vi "Climb Functions.vi"(6 "Elevator Slow Velocity":dbl=400.0, 9 "Elevator Slow Acceleration":dbl=800.0, 10 "POVs":i16[](array[numeric]), 11 "Buttons":bool[](array[boolean])) -> ()   [LabVIEW 2019]
uses:
  Typedef/XBox Buttons.ctl
  <vilib>/Rock Robotics/WPI/Solenoid/WPI_SolenoidValue.ctl
  <vilib>/Rock Robotics/WPI/ThirdParty/REV Robotics/SPARK MAX/Typedef/Spark MAX Idle Mode.ctl
  <vilib>/Rock Robotics/WPI/Solenoid/WPI_SolenoidSetEnum.vi
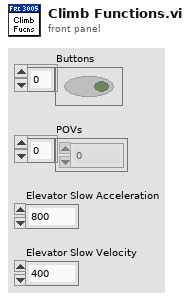
[diagram p1: front panel]
types:
  T1 = typedef "XBox Buttons.ctl" = enum16{"A", "B", "X", "Y", "Left Bumper", "Right Bumper", "Back", "Start", "Left Joystick", "Right Joystick"}
  T2 = typedef "Spark MAX Idle Mode.ctl" = enum16{"Coast", "Brake"}
  T3 = typedef "SPARKMAX6Motor.ctl" = cluster{"FrontLeftMaster":T4, "FrontLeftSlave1":T4, "FrontLeftSlave2":T4, "FrontRightMaster":T4, "FrontRightSlave1":T4, "FrontRightSlave2":T4}
  T4 = typedef "WPI_MotorControlDeviceRef.ctl" = cluster{"DeviceStatus":errorcluster, "Type":T5, "PWM":cluster{"PWM Channel":T6, "DeadBand":T7}, "CAN":cluster{"Device Number":u8, "SetOutput VI Ref":variant, "GetOutput VI Ref":variant, "Enable VI Ref":variant, "Disable VI Ref":variant, "Data":variant}, "Invert":bool, "DIO PWM":cluster{"PWM \"Enable\" Channel":T6, "DIOChannel":T8, "PWM Rate":dbl}}
  T5 = typedef "WPI_MotorControlType.ctl" = enum16{"PWM", "CAN", "DIO PWM"}
  T6 = typedef "FPGA_DIOPWMChannel.ctl" = enum8{"PWM 0", "PWM 1", "PWM 2", "PWM 3", "PWM 4", "PWM 5", "PWM 6", "PWM 7", "PWM 8", "PWM 9", "PWM MXP 0", "PWM MXP 1", "PWM MXP 2", "PWM MXP 3", "PWM MXP 4", "PWM MXP 5", "PWM MXP 6", "PWM MXP 7", "PWM MXP 8", "PWM MXP 9", "Invalid"}
  T7 = typedef "WPI_PWMDeadband.ctl" = cluster{"Name":string, "maxPositivePwm":i32, "minPositivePwm":i32, "centerPwm":i32, "maxNegativePwm":i32, "minNegativePwm":i32, "angularRange":u16}
  T8 = typedef "FPGA_DIOChannel.ctl" = enum8{"DIO 0", "DIO 1", "DIO 2", "DIO 3", "DIO 4", "DIO 5", "DIO 6", "DIO 7", "DIO 8", "DIO 9", "DIO MXP 0", "DIO MXP 1", "DIO MXP 2", "DIO MXP 3", "DIO MXP 4", "DIO MXP 5", "DIO MXP 6", "DIO MXP 7", "DIO MXP 8", "DIO MXP 9", "DIO MXP 10", "DIO MXP 11", "DIO MXP 12", "DIO MXP 13", "DIO MXP 14", "DIO MXP 15", "SPI Port CS1", "SPI Port CS2", "SPI Port CS3", "SPI Port MISO", "SPI Port MOSI", "Invalid"}
  T9 = typedef "WPI_SolenoidValue.ctl" = enum16{"Off", "On", "Forward", "Reverse"}
  T10 = typedef "WPI_SolenoidDevRef.ctl" = cluster{"DevStatus":errorcluster, "Pneumatics Control Module":u8, "Forward Solenoid Channel":T11, "Reverse Solenoid Channel":T11}
  T11 = typedef "WPI_SolenoidChannel.ctl" = enum8{"Solenoid 0", "Solenoid 1", "Solenoid 2", "Solenoid 3", "Solenoid 4", "Solenoid 5", "Solenoid 6", "Solenoid 7", "Invalid"}
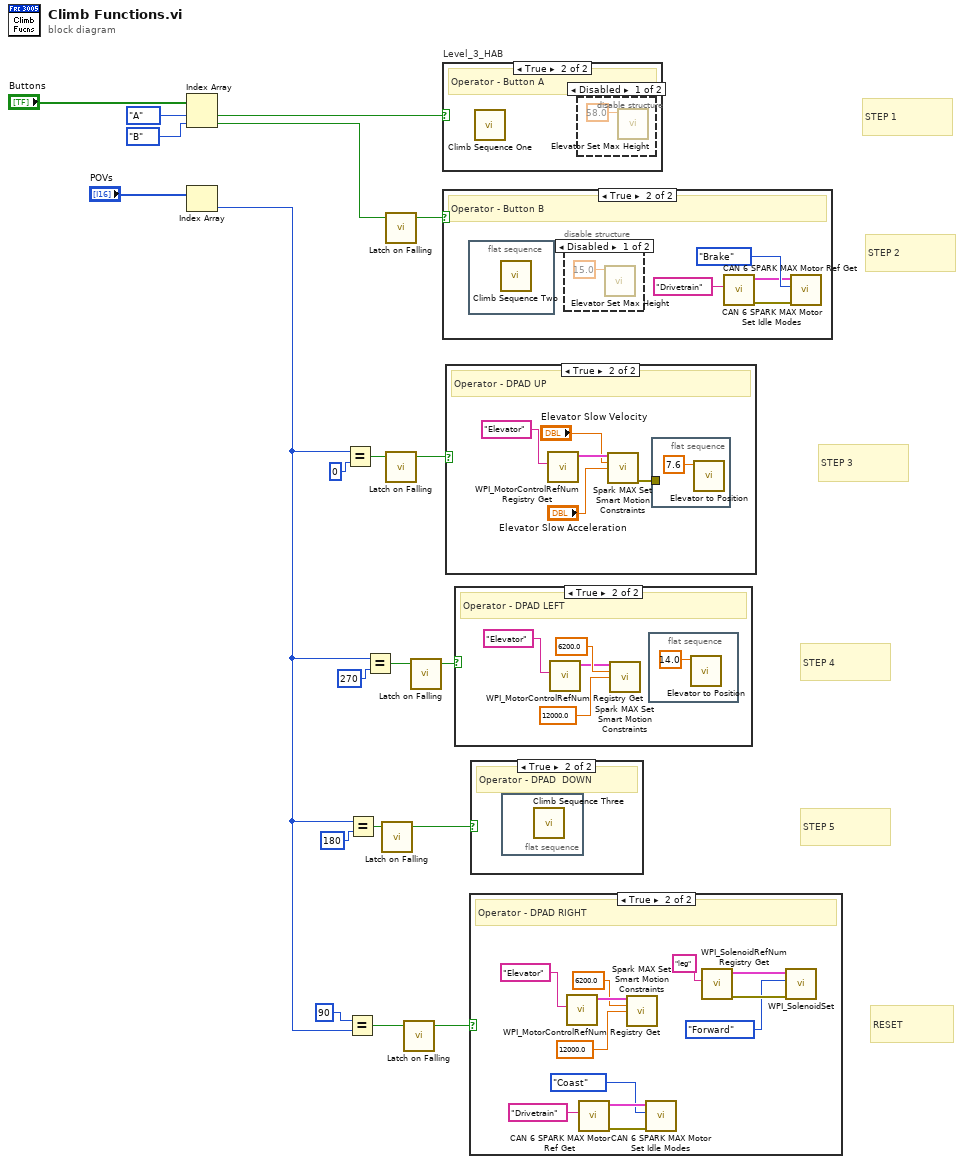
[diagram p0: block diagram]
diagram:
  # "RESET"
  # "STEP 5"
  # "STEP 4"
  # "STEP 3"
  # "STEP 2"
  # "STEP 1"
  n1 = Index Array(array="Buttons", index #1=XBox_Buttons."A" ("Enum"), index #2=XBox_Buttons."B" ("Enum")) -> (element #1=w20:bool, element #2=w19:bool)
  n2 = Index Array(array="POVs") -> (element=w15:i16)  [unwired: 1 in]
  n3 = Equal?(x=w15, y=i16 0 ("element")) -> (x = y?=w6:bool)
  n4 = Equal?(x=i16 90 ("element"), y=w15) -> (x = y?=w10:bool)
  n5 = Equal?(x=w15, y=i16 180 ("element")) -> (x = y?=w5:bool)
  n6 = Equal?(x=w15, y=i16 270 ("element")) -> (x = y?=w13:bool)
  n7 = call "Latch on Falling.vi"("Boolean in"=w5) -> ("Boolean out"=w2:bool)  [unwired: 4 in]
  n8 = call "Latch on Falling.vi"("Boolean in"=w19) -> ("Boolean out"=w3:bool)  [unwired: 4 in]
  n9 = call "Latch on Falling.vi"("Boolean in"=w6) -> ("Boolean out"=w8:bool)  [unwired: 4 in]
  n10 = call "Latch on Falling.vi"("Boolean in"=w10) -> ("Boolean out"=w11:bool)  [unwired: 4 in]
  n11 = call "Latch on Falling.vi"("Boolean in"=w13) -> ("Boolean out"=w14:bool)  [unwired: 4 in]
  n12 = case "Level_3_HAB" shown="True" w20 {
    frame False {
    }
    frame True {
      # "Operator - Button A"
      n13 = call "Climb Sequence One.vi"() -> ()  [unwired: 11 in, 1 out]
      n14 = disable-structure shown="Disabled" {
        frame Disabled {
          n15 = call "Elevator Set Max Height.vi"("Setpoint"=58.0) -> ()  [unwired: 10 in, 1 out]
        }
        frame Enabled {
        }
      }
    }
  }
  n16 = case shown="True" w3 {
    frame False {
    }
    frame True {
      # "Operator - Button B"
      n17 = flat-sequence {
        frame #0 {
          n18 = call "Climb Sequence Two.vi"() -> ()  [unwired: 11 in, 1 out]
        }
      }
      n19 = disable-structure shown="Disabled" {
        frame Disabled {
          n20 = call "Elevator Set Max Height.vi"("Setpoint"=15.0) -> ()  [unwired: 10 in, 1 out]
        }
        frame Enabled {
        }
      }
      n21 = call "CAN 6 SPARK MAX Motor Ref Get.vi"("refnum name"="Drivetrain") -> ("error out"=w22:errorcluster, "TalonSRX6MotorRef out"=w23:T3)  [unwired: 9 in]
      n22 = call "CAN 6 SPARK MAX Motor Set Idle Modes.vi"("error in (no error)"=w22, "Idle Mode"=Spark_MAX_Idle_Mode."Brake", "SPARK MAX ref in"=w23) -> ()  [unwired: 7 in, 2 out]
    }
  }
  n23 = case shown="True" w8 {
    frame False {
    }
    frame True {
      # "Operator - DPAD UP"
      n24 = call <vilib>:"WPI_MotorControlRefNum Registry Get.vi"("refnum name"="Elevator") -> ("MotorControlDevRef"=w31:T4)  [unwired: 9 in, 1 out]
      n25 = call <vilib>:"Spark MAX Set Smart Motion Constraints.vi"("MotorControlDeviceRef"=w31, "Max Velocity"="Elevator Slow Velocity", "Max Acceleration"="Elevator Slow Acceleration") -> ("error out"=w27:errorcluster)  [unwired: 11 in, 1 out]
      n26 = flat-sequence {
        tunnel: w27 -> [_]
        frame #0 {
          n27 = call "Elevator to Position.vi"("Elevator Height"=7.6) -> ()  [unwired: 10 in, 1 out]
        }
      }
    }
  }
  n28 = case shown="True" w14 {
    frame False {
    }
    frame True {
      # "Operator - DPAD LEFT"
      n29 = call <vilib>:"WPI_MotorControlRefNum Registry Get.vi"("refnum name"="Elevator") -> ("MotorControlDevRef"=w34:T4)  [unwired: 9 in, 1 out]
      n30 = call <vilib>:"Spark MAX Set Smart Motion Constraints.vi"("MotorControlDeviceRef"=w34, "Max Velocity"=6200.0, "Max Acceleration"=12000.0) -> ()  [unwired: 11 in, 2 out]
      n31 = flat-sequence {
        frame #0 {
          n32 = call "Elevator to Position.vi"("Elevator Height"=14.0) -> ()  [unwired: 10 in, 1 out]
        }
      }
    }
  }
  n33 = case shown="True" w11 {
    frame False {
    }
    frame True {
      # "Operator - DPAD RIGHT"
      n34 = call <vilib>:"WPI_MotorControlRefNum Registry Get.vi"("refnum name"="Elevator") -> ("MotorControlDevRef"=w48:T4)  [unwired: 9 in, 1 out]
      n35 = call "CAN 6 SPARK MAX Motor Ref Get.vi"("refnum name"="Drivetrain") -> ("error out"=w45:errorcluster, "TalonSRX6MotorRef out"=w44:T3)  [unwired: 9 in]
      n36 = call <vilib>:"Spark MAX Set Smart Motion Constraints.vi"("MotorControlDeviceRef"=w48, "Max Velocity"=6200.0, "Max Acceleration"=12000.0) -> ()  [unwired: 11 in, 2 out]
      n37 = call "CAN 6 SPARK MAX Motor Set Idle Modes.vi"("error in (no error)"=w45, "Idle Mode"=Spark_MAX_Idle_Mode."Coast", "SPARK MAX ref in"=w44) -> ()  [unwired: 7 in, 2 out]
      n38 = call <vilib>:"WPI_SolenoidRefNum Registry Get.vi"("refnum name"="leg") -> ("error out"=w39:errorcluster, "SolenoidDevRef"=w41:T10)  [unwired: 9 in]
      n39 = call-poly <vilib>:"WPI_SolenoidSet.vi"("error in (no error)"=w39, "Value"=WPI_SolenoidValue."Forward", "SolenoidDevRef"=w41) -> ()  [unwired: 7 in, 2 out]
    }
  }
  n40 = case shown="True" w2 {
    frame False {
    }
    frame True {
      # "Operator - DPAD  DOWN"
      n41 = flat-sequence {
        frame #0 {
          n42 = call "Climb Sequence Three.vi"() -> ()  [unwired: 11 in, 1 out]
        }
      }
    }
  }
